vi "Read P.vi"(8 "error in (no error)":errorcluster, 11 "Change PID Controls MSG in":refnum<class "Change PID Controls MSG.lvclass">) -> (0 "error out":errorcluster, 2 "P":dbl, 3 "Change PID Controls MSG out":refnum<class "Change PID Controls MSG.lvclass">)   [LabVIEW 2014, in "Change PID Controls MSG.lvclass"]
uses:
  Change PID Controls MSG.lvclass
  Change PID Controls MSG.lvclass/Change PID Controls MSG.ctl
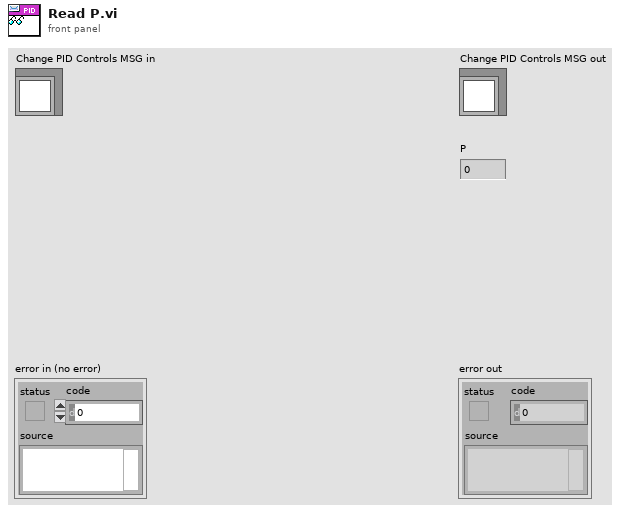
[diagram p1: front panel]
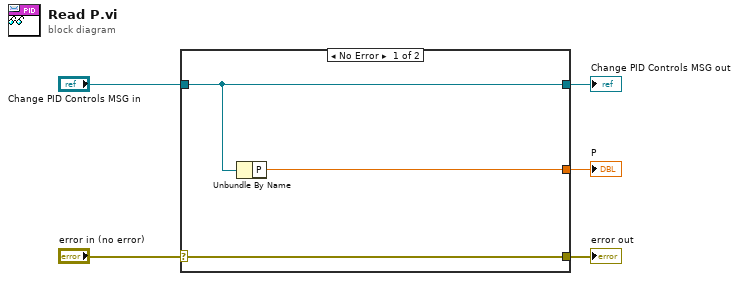
[diagram p0: block diagram]
diagram:
  n1 = case shown="No Error" "error in (no error)" {
    selector: "error in (no error)" -> [w8 w9]
    tunnel: [w8 w9] -> w4
    tunnel: [w7 w10] -> w2
    tunnel: "Change PID Controls MSG in" -> [w7 w10]
    tunnel: [w6 _] -> w1
    frame No Error {
      n2 = Unbundle By Name(w7) -> ("P"=w6:dbl)
    }
    frame Error {
    }
  }
  "error out" <- w4
  "Change PID Controls MSG out" <- w2
  "P" <- w1
